vi "oa_Trigger Limit Range.vi"(0 "processing mode":u16(ring) items=["Continuous", "Compute at Time Interval", "Compute at Speed Interval"], 5 "Limit range":bool, 7 "steps input":cluster{"start":dbl, "end":dbl, "step":dbl} {"step" format="%.2f"; "end" format="%.2f"; "start" format="%.2f"}, 11 "error in (no error)":errorcluster) -> (4 "processing mode duplicate":u16, 8 "steps output":cluster{"start":dbl, "end":dbl, "step":dbl}, 15 "error out":errorcluster)   [LabVIEW 2017, in "SoundVib_OAUtility.lvlib"]
uses:
  <vilib>/addons/Sound and Vibration/Order Analysis/Utility/SoundVib_OAUtility.lvlib
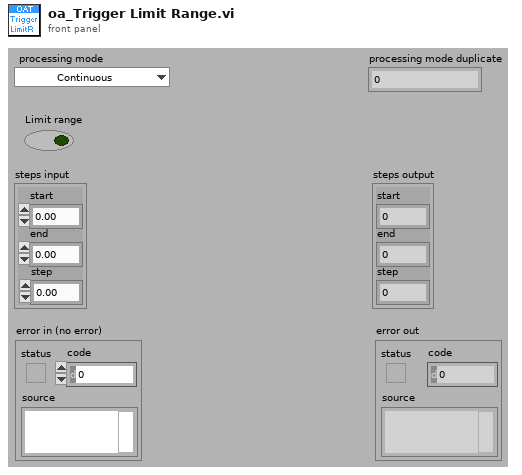
[diagram p1: front panel]
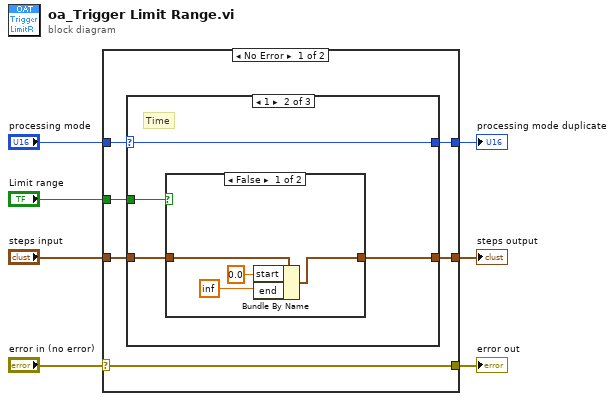
[diagram p0: block diagram]
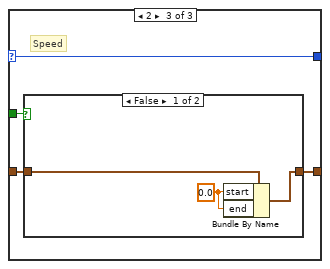
[diagram p4: hidden frame]
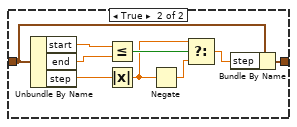
[diagram p5: hidden frame]
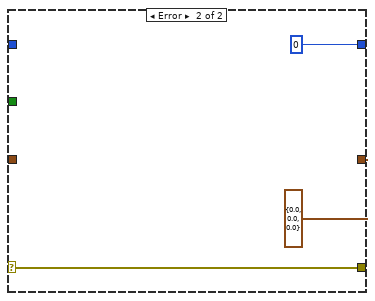
[diagram p6: hidden frame]
diagram:
  n1 = case shown="No Error" "error in (no error)" {
    selector: "error in (no error)" -> [w8 w41]
    tunnel: "processing mode" -> [w13 _]
    tunnel: [w12 u16 0 ("processing mode")] -> w5
    tunnel: [w11 cluster{"start":dbl, "end":dbl, "step":dbl} {"start"=0.0, "end"=0.0, "step"=0.0} ("steps input")] -> w4
    tunnel: "steps input" -> [w10 _]
    tunnel: "Limit range" -> [w9 _]
    tunnel: [w8 w41] -> w1
    frame No Error {
      n2 = case shown="1" w13 {
        selector: w13 -> [w15 w19 w28]
        tunnel: [w15 w19 w28] -> w12
        tunnel: [w14 w16 w26] -> w11
        tunnel: w10 -> [w14 w17 w27]
        tunnel: w9 -> [_ w18 w25]
        frame 0, Default {
        }
        frame 1 {
          # "Time"
          n3 = case shown="False" w18 {
            tunnel: w17 -> [w23 w24]
            tunnel: [w20 w24] -> w16
            frame False {
              n4 = Bundle By Name(cluster=w23, "start"=0.0, "end"=inf) -> (w20:cluster{"start":dbl, "end":dbl, "step":dbl})
            }
            frame True {
            }
          }
        }
        frame 2 {
          # "Speed"
          n5 = case shown="False" w25 {
            tunnel: w27 -> [w31 w34]
            tunnel: [w29 w32] -> w26
            frame False {
              w30 = 0.0 ("start")
              n6 = Bundle By Name(cluster=w31, "start"=w30, "end"=w30) -> (w29:cluster{"start":dbl, "end":dbl, "step":dbl})
            }
            frame True {
              n7 = Unbundle By Name(w34) -> ("start"=w40:dbl, "end"=w39:dbl, "step"=w37:dbl)
              n8 = Less Or Equal?(x=w40, y=w39) -> (x <= y?=w38:bool)
              n9 = Absolute Value(x=w37) -> (abs(x)=w36:dbl)
              n10 = Negate(x=w36) -> (-x=w35:dbl)
              n11 = Select(t=w36, s=w38, f=w35) -> (s? t:f=w33:dbl)
              n12 = Bundle By Name(cluster=w34, "step"=w33) -> (w32:cluster{"start":dbl, "end":dbl, "step":dbl})
            }
          }
        }
      }
    }
    frame Error {
    }
  }
  "error out" <- w1
  "steps output" <- w4
  "processing mode duplicate" <- w5
